vi "refMgr_Example1.vi"() -> ()   [LabVIEW 2017]
uses:
  RefManager/TagDB RefManager.lvlib
  <userlib>/_NEVSTOP/TagDB/TagDB.lvlib
panel:
  out "::DB items::":string[](array[string])
  in  "Tab Control":enum32{"Page 1", "Page 2", "Page 3"}(tab)
  out "Waveform Chart 2":dbl(graph)
  out "Waveform Chart 3":dbl(graph)
  out "Waveform Chart 1":dbl(graph)
  in  "Combo Box":string(combo)
  out "error out":errorcluster
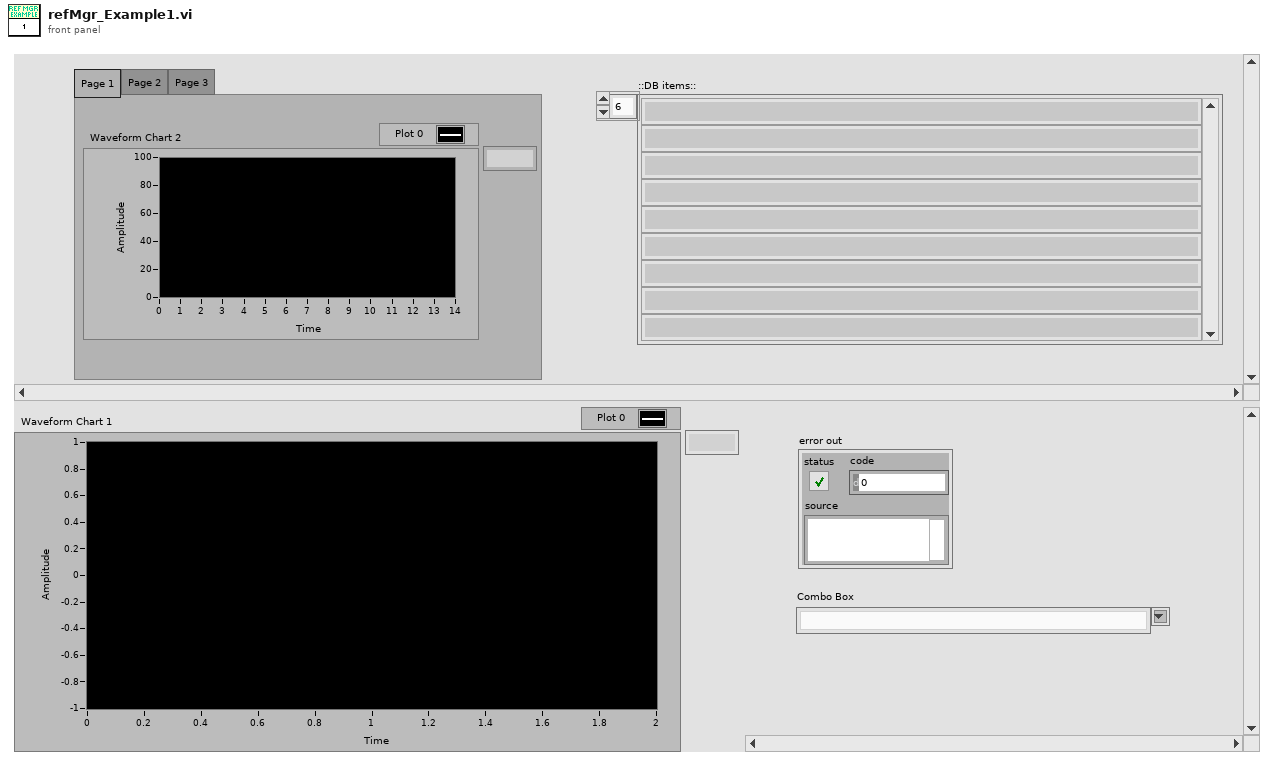
[diagram p1: front panel]
types:
  T1 = typedef "TagDB.lvlib/TagDB.ctl" = refnum<k1>
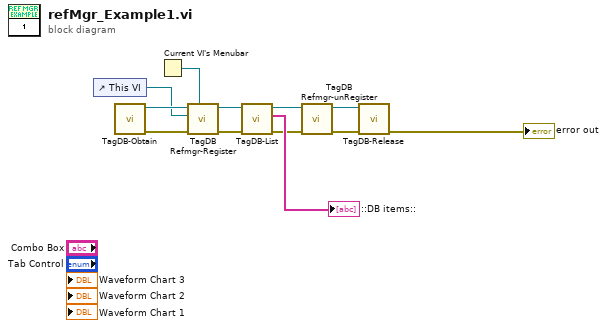
[diagram p0: block diagram]
diagram:
  n1 = control-ref of="This VI"() -> (w2:refnum<vi>)
  n2 = call <userlib>:"TagDB-Obtain.vi"() -> ("error out"=w9:errorcluster, "TagDB"=w11:T1)  [unwired: 5 in, 1 out]
  n3 = Current VI's Menubar() -> (w1:refnum<k9>)
  n4 = call "TagDB Refmgr-Register.vi"("menu reference"=w1, "error in (no error)"=w9, "VI Refnum"=w2, "TagDB in"=w11) -> ("error out"=w7:errorcluster, "TagDB out"=w10:T1)  [unwired: 5 in, 1 out]
  n5 = call <userlib>:"TagDB-List.vi"("error in (no error)"=w7, "TagDB"=w10) -> ("error out"=w4:errorcluster, "names"=→"::DB items::":string[], "TagDB(dup)"=w8:T1)  [unwired: 6 in, 1 out]
  n6 = call "TagDB Refmgr-unRegister.vi"("error in (no error)"=w4, "TagDB in"=w8) -> ("error out"=w3:errorcluster, "TagDB out"=w5:T1)  [unwired: 8 in]
  n7 = call <userlib>:"TagDB-Release.vi"("error in (no error)"=w3, "TagDB"=w5) -> ("error out"=→"error out":errorcluster)  [unwired: 9 in]
